vi "Find control ref.vi"(8 "error in (no error)":errorcluster, 10 "Label":string="Parameters", 11 "Controls[]":refnum<vi>[](array[refnum])) -> (0 "error out":errorcluster, 2 "Found":bool, 3 "Control out":refnum<vi>)   [LabVIEW 2015, in "Mag Lab Measure UI.lvclass"]
uses:
  Mag Lab Measure UI.lvclass
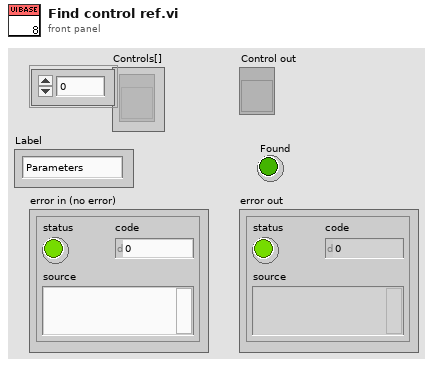
[diagram p1: front panel]
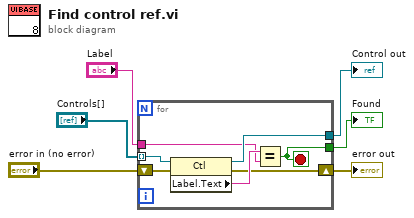
[diagram p0: block diagram]
diagram:
  n1 = for {
    tunnel: "Controls[]" -> [w12] mode=indexing
    tunnel: [w10] -> w5
    tunnel: [w9] -> w6
    shift-right: [w8] -> w4
    shift-left: "error in (no error)" -> [w13]
    tunnel: "Label" -> [w7]
    stop <- w10 stop-if-true
    n2 = property class="Ctl"(reference=w12, error in=w13) -> (reference out=w9:refnum<vi>, error out=w8:errorcluster, "Label.Text"=w11:string)
    n3 = Equal?(x=w11, y=w7) -> (x = y?=w10:bool)
  }
  "Control out" <- w6
  "Found" <- w5
  "error out" <- w4
